vi "FindCam.vi"(8 "error in (no error)":errorcluster) -> (0 "error out":errorcluster, 3 "cameraFound":bool)   [LabVIEW 2015, in "ESLSCDLL.lvlib"]
uses:
  ESLSCDLL.lvlib
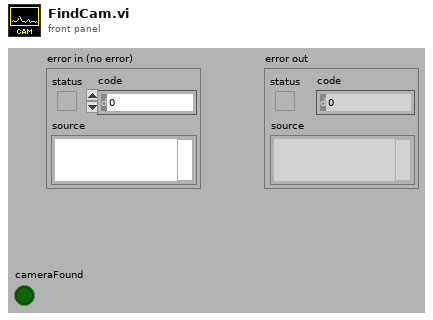
[diagram p1: front panel]
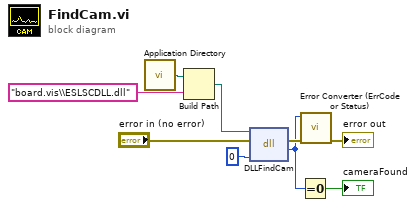
[diagram p0: block diagram]
diagram:
  n1 = call <vilib>:"Application Directory.vi"() -> ("Application Directory"=w6:path)
  n2 = Build Path(base path=w6, name or relative path="board.vis\\ESLSCDLL.dll") -> (appended path=w4:path)
  n3 = dll-call lib="C:/ENTW/PCIE/LV64/board.vis/ESLSCDLL.dll" fn="DLLFindCam" ("lwlscdll.dll:DLLWriteLongS0")(path in=w4, error in="error in (no error)", "drvno"=u32 0) -> (error out=w7:errorcluster, "es_status_codes"=w1:i32)  [unwired: 2 in, 1 out]
  n4 = Equal To 0?(x=w1) -> (x = 0?=→"cameraFound":bool)
  n5 = call "Error Converter (ErrCode or Status).vi"("error in (no error)"=w7, "error code"=w1) -> ("error out"=→"error out":errorcluster)  [unwired: 9 in]
